vi "UniqueID2Data.vi"(11 "UniqueID":string) -> (3 "Data":string)   [LabVIEW 2013]
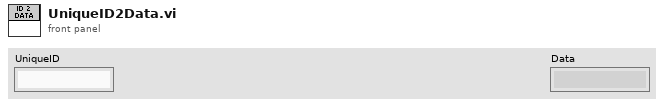
[diagram p1: front panel]
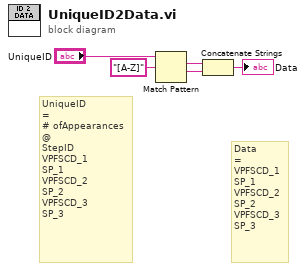
[diagram p0: block diagram]
diagram:
  # "Data\n=\nVPFSCD_1\nSP_1\nVPFSCD_2\nSP_2\nVPFSCD_3\nSP_3"
  # "UniqueID\n=\n# ofAppearances\n@\nStepID\nVPFSCD_1\nSP_1\nVPFSCD_2\nSP_2\nVPFSCD_3\nSP_3"
  n1 = Match Pattern(string="UniqueID", regular expression="[A-Z]") -> (match substring=w3:string, after substring=w2:string)  [unwired: 1 in, 2 out]
  n2 = Concatenate Strings(w3, w2) -> (→"Data":string)
